vi "testExecutionView.vi"() -> ()   [LabVIEW 2015, in "ILCBTViews.lvlib"]
uses:
  ILCBTViews.lvlib
  UserEvents/UserEvents.lvclass
  UserEvents/UserEvents.lvclass/UserEvents.ctl
  Typedefs/StateSelector.ctl
  Commands/StartTestScenarioCommand/StartTestScenarioCommand.lvclass
  abortTestSeries.vi
  Typedefs/ILCBTTypedefs.lvlib
panel:
  in  "Comments":string
  in  "Operator":string
  in  "Serial Number":string
  in  "executeAllTests?":bool
  in  "UserEvents in":refnum<class "UserEvents.lvclass">
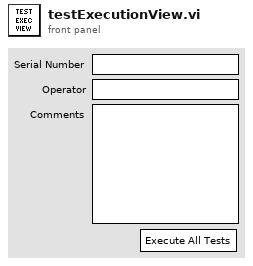
[diagram p1: front panel]
types:
  T1 = typedef "ILCBTTypedefs.lvlib/PubDataEvents.ctl" = cluster{"State":refnum<user-event>, "ErrorCode":refnum<user-event>, "OutputData":refnum<user-event>, "LogPath":refnum<user-event>, "TestScenarioCompleted":refnum<user-event>, "TestScenarioStarted":refnum<user-event>, "TestingStarted":refnum<user-event>, "StartTestScenario":refnum<user-event>}
  T2 = typedef "ILCBTTypedefs.lvlib/SubDataEvents.ctl" = cluster{"Command":refnum<user-event>}
  T3 = cluster{"Event Registration Refnum":refnum<event-registration>}
  T4 = typedef "ILCBTTypedefs.lvlib/StateSelector.ctl" = enum16{"EnabledState", "FaultState", "OffState", "StandbyState", "WaitingForTestState", "ExecutingTestState"}
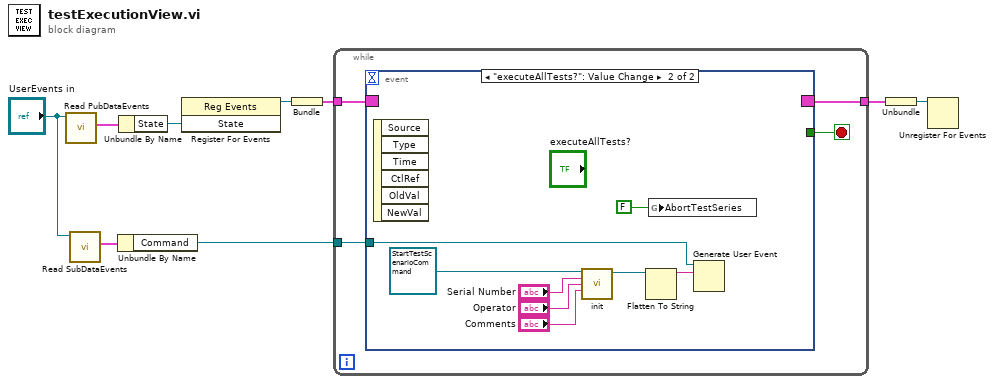
[diagram p0: block diagram]
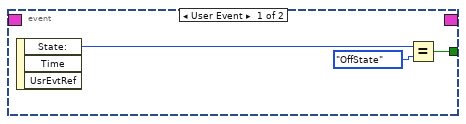
[diagram p2: hidden frame]
diagram:
  n1 = call "Read PubDataEvents.vi"("UserEvents in"="UserEvents in") -> ("PubDataEvents"=w9:T1)  [unwired: 9 in, 1 out]
  n2 = call "Read SubDataEvents.vi"("UserEvents in"="UserEvents in") -> ("SubDataEvents"=w2:T2)  [unwired: 9 in, 1 out]
  n3 = Unbundle By Name(w2) -> ("Command"=w1:refnum<user-event>)
  n4 = Unbundle By Name(w9) -> ("State"=w8:refnum<user-event>)
  n5 = register-events(w8) -> (reference out=w7:refnum<event-registration>)  [unwired: 2 in, 1 out]
  n6 = Bundle("Event Registration Refnum"=w7) -> (w6:T3)  [unwired: 1 in]
  n7 = while {
    tunnel: w6 -> [w10]
    tunnel: [w11] -> w5
    tunnel: w1 -> [w12]
    stop <- w13 stop-if-true
    n8 = event shown="[1] \"executeAllTests?\": Value Change" {
      selector: w10 -> [_ _]
      dyn-events: [_ _] -> w11
      timeout: _ -> [_ _]
      tunnel: [w15 _] -> w13
      tunnel: w12 -> [_ w23]
      event User Event {
        n9 = event-data() -> ("State:"=w14:T4)  [unwired: 1 in, 2 out]
        n10 = Equal?(x=w14, y=StateSelector."OffState" ("State:")) -> (x = y?=w15:bool)
      }
      event "executeAllTests?": Value Change {
        n11 = event-data() -> ()  [unwired: 1 in, 6 out]
        n12 = call "init.vi"("StartTestScenarioCommand in"=refnum<class "StartTestScenarioCommand.lvclass"> refnum ("StartTestScenarioCommand.lvclass"), "Serial Number"="Serial Number", "Operator"="Operator", "Comments"="Comments") -> ("StartTestScenarioCommand out"=w21:refnum<class "StartTestScenarioCommand.lvclass">)  [unwired: 10 in, 1 out]
        n13 = Flatten To String(anything=w21) -> (data string=w24:string)  [unwired: 3 in, 2 out]
        n14 = global write "abortTestSeries.vi" "AbortTestSeries"(FALSE ("AbortTestSeries")) -> ()
        n15 = Generate User Event(user event=w23, event data cluster=w24) -> ()  [unwired: 2 in, 2 out]
      }
    }
  }
  n16 = Unbundle(w5) -> ("Event Registration Refnum"=w4:refnum<event-registration>)
  n17 = Unregister For Events(event registration refnum=w4) -> ()  [unwired: 1 in, 1 out]
